vi "GetSystemsInfo.vi"() -> (0 "Pos Info":T1)   [LabVIEW 2015]
uses:
  Sherman/Desktop/BETA_GSCS/Systems/Coll_Focus/GSP_COLL_Global.vi
  Sherman/Desktop/BETA_GSCS/Systems/Grating_Translation/GSP_GT_Global.vi
  Sherman/Desktop/BETA_GSCS/Systems/Primary Filter/GSP_F1_Global.vi
  Sherman/Desktop/BETA_GSCS/Systems/Secondary Filter/GSP_F2_Global.vi
  Sherman/Desktop/BETA_GSCS/Systems/Slit/GSP_SLIT_Global.vi
  GSCS Scripting/Utils/GSP_Wavelength_Global.vi
  Sherman/Desktop/BETA_GSCS/Systems/Cam_Focus/GSP_CF_Global.vi
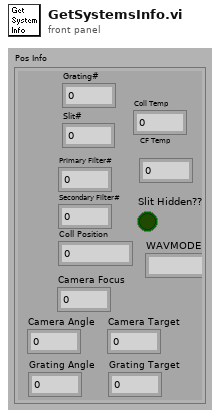
[diagram p1: front panel]
types:
  T1 = cluster{"Grating#":i32, "Slit#":i32, "Primary Filter#":i32, "Secondary Filter#":i32, "Coll Position":i32, "Camera Focus":i32, "Camera Angle":dbl, "Grating Angle":dbl, "Coll Temp":dbl, "CF Temp\n":dbl, "Camera Target":dbl, "Grating Target":dbl, "WAVMODE":string, "Slit Hidden??":bool}
  T2 = cluster{"Grating#":i32, "Slit#":i32, "Primary Filter#":i32, "Secondary Filter#":i32, "Coll Position":i32, "Camera Focus":i32, "Camera Angle":dbl, "Grating Angle":dbl, "Coll Temp":dbl, "CF Temp":dbl, "Camera Target":dbl, "Grating Target":dbl, "WAVMODE":string, "Slit Hidden?":bool}
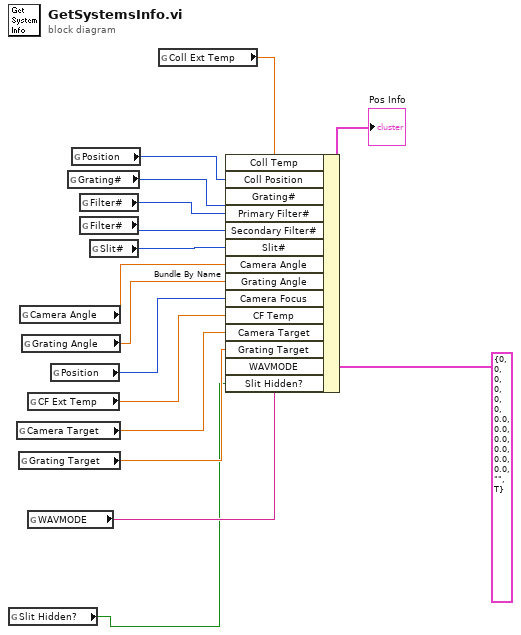
[diagram p0: block diagram]
diagram:
  n1 = global read "GSP_SLIT_Global.vi" "Slit Hidden?"() -> (w1:bool)
  n2 = global read "GSP_Wavelength_Global.vi" "Camera Target"() -> (w4:dbl)
  n3 = global read "GSP_Wavelength_Global.vi" "Grating Target"() -> (w3:dbl)
  n4 = global read "GSP_Wavelength_Global.vi" "Camera Angle"() -> (w11:dbl)
  n5 = global read "GSP_Wavelength_Global.vi" "Grating Angle"() -> (w10:dbl)
  n6 = global read "GSP_CF_Global.vi" "CF Ext Temp"() -> (w6:dbl)
  n7 = global read "GSP_Wavelength_Global.vi" "WAVMODE"() -> (w2:string)
  n8 = global read "GSP_CF_Global.vi" "Position"() -> (w9:i32)
  n9 = global read "GSP_GT_Global.vi" "Grating#"() -> (w12:i32)
  n10 = global read "GSP_COLL_Global.vi" "Position"() -> (w16:i32)
  n11 = global read "GSP_F1_Global.vi" "Filter#"() -> (w15:i32)
  n12 = global read "GSP_F2_Global.vi" "Filter#"() -> (w14:i32)
  n13 = global read "GSP_SLIT_Global.vi" "Slit#"() -> (w13:i32)
  n14 = global read "GSP_SLIT_Global.vi" "Coll Ext Temp"() -> (w5:dbl)
  n15 = Bundle By Name(cluster=T2 {"Grating#"=0, "Slit#"=0, "Primary Filter#"=0, "Secondary Filter#"=0, "Coll Position"=0, "Camera Focus"=0, "Camera Angle"=0.0, "Grating Angle"=0.0, "Coll Temp"=0.0, "CF Temp"=0.0, "Camera Target"=0.0, "Grating Target"=0.0, "WAVMODE"="", "Slit Hidden?"=TRUE} ("Pos Info"), "Coll Temp"=w5, "Coll Position"=w16, "Grating#"=w12, "Primary Filter#"=w15, "Secondary Filter#"=w14, "Slit#"=w13, "Camera Angle"=w11, "Grating Angle"=w10, "Camera Focus"=w9, "CF Temp"=w6, "Camera Target"=w4, "Grating Target"=w3, "WAVMODE"=w2, "Slit Hidden?"=w1) -> (→"Pos Info":T2)
